vi "searchElement.vi"(8 "input":cluster{"name":string, "type desc":i16[]}[](array[cluster]), 11 "name":string) -> (3 "output":cluster{"name":string, "type desc":i16[]})   [LabVIEW 2010]
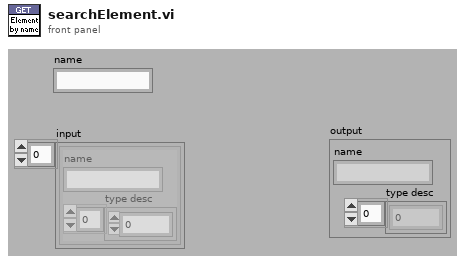
[diagram p1: front panel]
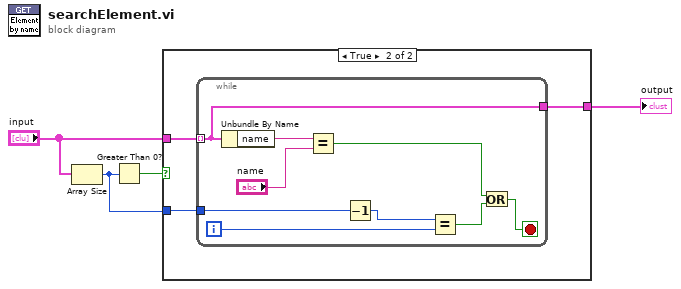
[diagram p0: block diagram]
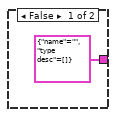
[diagram p2: hidden frame]
diagram:
  n1 = Array Size(array="input") -> (size(s)=w2:i32)
  n2 = Greater Than 0?(x=w2) -> (x > 0?=w4:bool)
  n3 = case shown="True" w4 {
    tunnel: "input" -> [_ w8]
    tunnel: w2 -> [_ w7]
    tunnel: [cluster{"name":string, "type desc":i16[]} {"name"="", "type desc"=[]} w6] -> w1
    frame False {
    }
    frame True {
      n4 = while {
        tunnel: w8 -> [w9] mode=indexing
        tunnel: w7 -> [w12]
        tunnel: [w9] -> w6
        i -> [w13]
        stop <- w15 stop-if-true
        n5 = Unbundle By Name(w9) -> ("name"=w17:string)
        n6 = Equal?(x=w17, y="name") -> (x = y?=w14:bool)
        n7 = Decrement(x=w12) -> (x-1=w11:i32)
        n8 = Equal?(x=w11, y=w13) -> (x = y?=w10:bool)
        n9 = Or(x=w14, y=w10) -> (x .or. y?=w15:bool)
      }
    }
  }
  "output" <- w1
